vi "Query Status Register.vi"(8 "error in":errorcluster, 11 "6032A in":refnum<class "6032A.lvclass">) -> (0 "error out":errorcluster, 3 "6032A out":refnum<class "6032A.lvclass">)   [LabVIEW 2019, in "6032A.lvlib" / "6032A.lvclass"]
doc: "Child classes must override this VI:\n\nThis VI is the device specific query of the supply's status registers. \nThe return values are: \n\nThe implementation must read status registers and push the status register values to private data for:\nOCP Flag, OVP Flag, Interlock Flag, Output Flag into the private data arrays of the power supply class."
uses:
  Library/6032A.lvclass
  C:/Users/Public/Documents/Development/builds/Instruments/PowerSupply.lvlibp/Library/PowerSupply.lvclass
  builds/Instruments/PowerSupply.lvlibp/Custom Controls/Status_Flags.ctl
  builds/Instruments/PowerSupply.lvlibp/Accessors/Write Status Flags.vi
  builds/Instruments/PowerSupply.lvlibp/Library/PowerSupply.lvclass
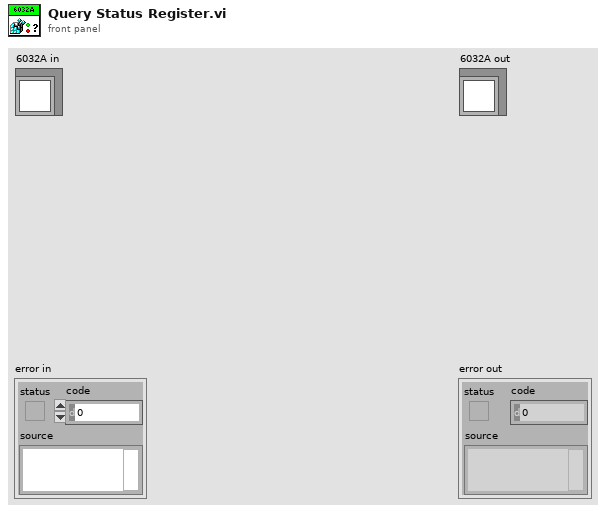
[diagram p1: front panel]
types:
  T1 = typedef "PowerSupply.lvlibp/PowerSupply.lvclass/Status_Flags.ctl" = cluster{"Interlock":bool, "OVP":bool, "OCP":bool, "Output":bool}
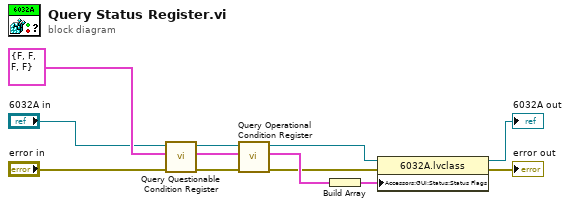
[diagram p0: block diagram]
diagram:
  n1 = call "Query Questionable Condition Register.vi"("error in"="error in", "Status in"=T1 {"Interlock"=FALSE, "OVP"=FALSE, "OCP"=FALSE, "Output"=FALSE} ("Status"), "6032A in"="6032A in") -> ("error out"=w4:errorcluster, "Status out"=w6:T1, "6032A out"=w5:refnum<class "6032A.lvclass">)  [unwired: 6 in]
  n2 = call "Query Operational Condition Register.vi"("error in"=w4, "Status in"=w6, "6032A in"=w5) -> ("error out"=w1:errorcluster, "Status out"=w2:T1, "6032A out"=w3:refnum<class "6032A.lvclass">)  [unwired: 6 in]
  n3 = Build Array(w2) -> (w10:T1[])
  n4 = property class="6032A.lvclass"(reference=w3, error in=w1, "Accessors:GUI:Status:Status Flags"=w10) -> (reference out=→"6032A out":refnum<class "6032A.lvclass">, error out=→"error out":errorcluster)
